vi "Find Project Test Objects.vi"(8 "error in":errorcluster, 10 "Project":path) -> (0 "error out":errorcluster, 2 "TestPaths":path[](array[path]))   [LabVIEW 2011, in "VITesterUtilities.lvlib"]
uses:
  Libraries/VITesterUtilities.lvlib
  <userlib>/_OpenG.lib/array/array.llb/Conditional Auto-Indexing Tunnel (Path)__ogtk.vi
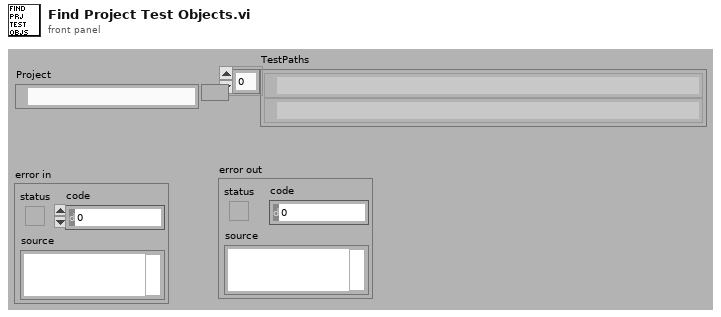
[diagram p1: front panel]
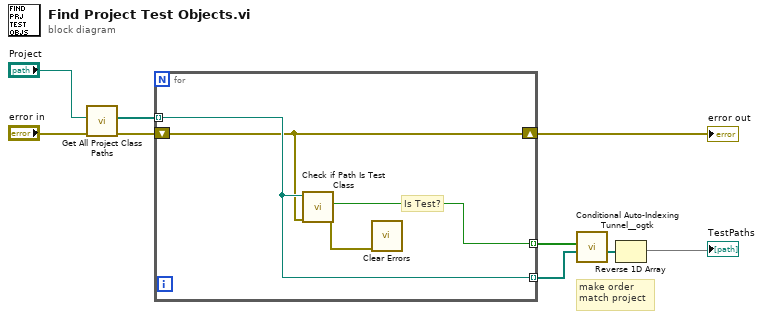
[diagram p0: block diagram]
diagram:
  # "make order\nmatch project"
  n1 = call "Get All Project Class Paths.vi"("error in"="error in", "Project File"="Project") -> ("error out"=w3:errorcluster, "Project Classes"=w1:path[])  [unwired: 8 in]
  n2 = for {
    shift-right: [w10] -> w6
    shift-left: w3 -> [w10]
    tunnel: [w11] -> w8 mode=indexing
    tunnel: [w13] -> w5 mode=indexing
    tunnel: w1 -> [w11] mode=indexing
    # "Is Test?"
    n3 = call "Check if Path Is Test Class.vi"("error in"=w10, "Test Class Path"=w11) -> ("error out"=w12:errorcluster, "IsTestObject"=w13:bool)  [unwired: 7 in, 1 out]
    n4 = call <vilib>:"Clear Errors.vi"("error in (no error)"=w12) -> ()  [unwired: 6 in, 1 out]
  }
  "error out" <- w6
  n5 = call-poly <userlib>:"Conditional Auto-Indexing Tunnel__ogtk.vi"("Array in"=w8, "Elements to keep"=w5) -> ("Filtered Array out"=w7:path[])  [unwired: 5 in]
  n6 = Reverse 1D Array(array=w7) -> (reversed array=→"TestPaths":path[])
